vi "7_1_Recursivefunc.vi"(6 "disabled index (col)":i32, 9 "Hands(objs) to look at":i32[](array[numeric]), 10 "Rank":i32, 11 "Array in":refnum<class "CardHand.lvclass">[](array[class])) -> (3 "Array out":refnum<class "CardHand.lvclass">[](array[class]), 5 "Rank 2":i32)   [LabVIEW 2021, in "2023.lvlib"]
uses:
  2023.lvlib
  CardHand.lvclass
  CardHand.lvclass/CardHand.ctl
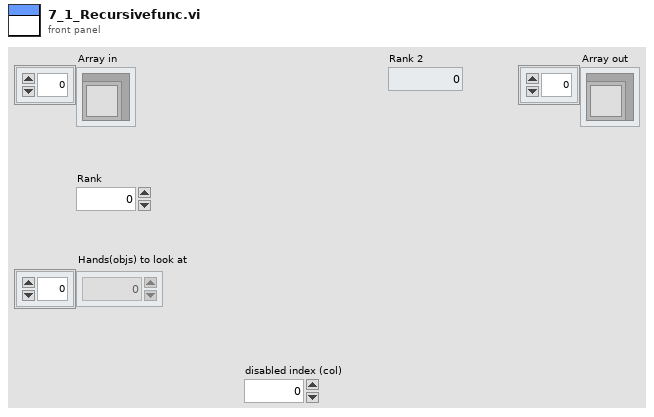
[diagram p1: front panel]
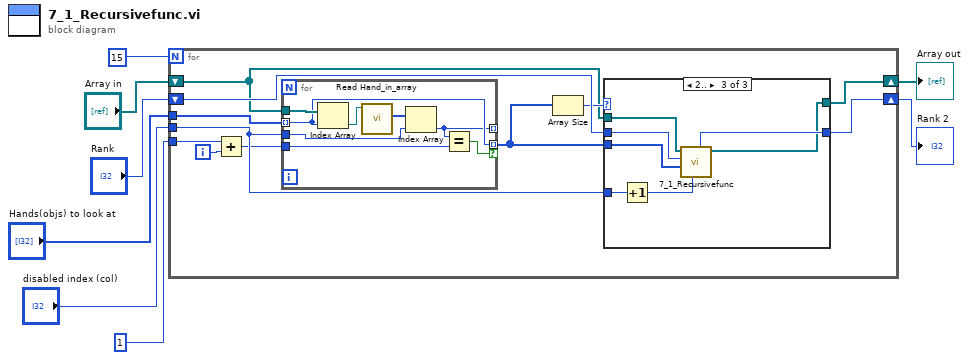
[diagram p0: block diagram]
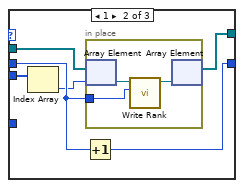
[diagram p3: hidden frame]
diagram:
  n1 = for {
    N: 15 ("y") -> [_]
    shift-right: [w17] -> w5
    shift-left: "Array in" -> [w13]
    shift-right: [w14] -> w3
    shift-left: "Rank" -> [w16]
    tunnel: 1 ("x") -> [w18]
    tunnel: "disabled index (col)" -> [w11]
    tunnel: "Hands(objs) to look at" -> [w12]
    i -> [w19]
    n2 = Add(x=w18, y=w19) -> (x+y=w10:i32)
    n3 = for {
      tunnel: w13 -> [w27]
      tunnel: w12 -> [w23] mode=indexing
      tunnel: w11 -> [w24]
      tunnel: [w21] -> _ mode=indexing
      tunnel: [w23] -> w9 mode=indexing if=w20
      tunnel: w10 -> [w22]
      n4 = Index Array(array=w27, index=w23) -> (element=w26:refnum<class "CardHand.lvclass">)
      n5 = call "Read Hand_in_array.vi"("CardHand in"=w26) -> ("Hand_in_array"=w25:i32[])  [unwired: 8 in, 2 out]
      n6 = Index Array(array=w25, index=w24) -> (element=w21:i32)
      n7 = Equal?(x=w21, y=w22) -> (x = y?=w20:bool)
    }
    n8 = Array Size(array=w9) -> (size(s)=w15:i32)
    n9 = case shown="2.." w15 {
      tunnel: [w29 w32 w39] -> w17
      tunnel: w16 -> [w28 w35 w45]
      tunnel: w13 -> [w29 w33 w41]
      tunnel: [w28 w34 w42] -> w14
      tunnel: w11 -> [_ _ w44]
      tunnel: w9 -> [_ w30 w40]
      frame 0, Default {
      }
      frame 1 {
        n10 = Index Array(array=w30) -> (element=w31:i32)  [unwired: 1 in]
        n11 = Increment(x=w35) -> (x+1=w34:i32)
        n12 = in-place {
          in-place-border: w35 -> [w36]
          n13 = in-place-array #1(w33, w31) -> (w38:refnum<class "CardHand.lvclass">)
          n14 = call "Write Rank.vi"("Rank"=w36, "CardHand in"=w38) -> ("CardHand out"=w37:refnum<class "CardHand.lvclass">)  [unwired: 8 in, 1 out]
          n15 = in-place-array #1(w37) -> (w32:refnum<class "CardHand.lvclass">[])  [unwired: 1 out]
        }
      }
      frame 2.. {
        n16 = Increment(x=w44) -> (x+1=w43:i32)
        n17 = call "7_1_Recursivefunc.vi"("disabled index (col)"=w43, "Hands(objs) to look at"=w40, "Rank"=w45, "Array in"=w41) -> ("Array out"=w39:refnum<class "CardHand.lvclass">[], "Rank 2"=w42:i32)  [unwired: 6 in]
      }
    }
  }
  "Array out" <- w5
  "Rank 2" <- w3
